vi "UpperMidbrain.vi"(5 "Boat Heading":dbl, 6 "tweak":T2, 7 "WhatAroundMeMap?":cluster{"T":dbl, "Range":dbl, "Bearing":dbl}[](array[cluster]), 8 "SOFT E-STOP":bool, 9 "behavior weights":i8[](array[numeric])=[0, 1, 0], 10 "ir distance":i32, 11 "ForeBrain to Midbrain":T1) -> (3 "string":string)   [LabVIEW 2012]
panel:
  # "under cloud?"
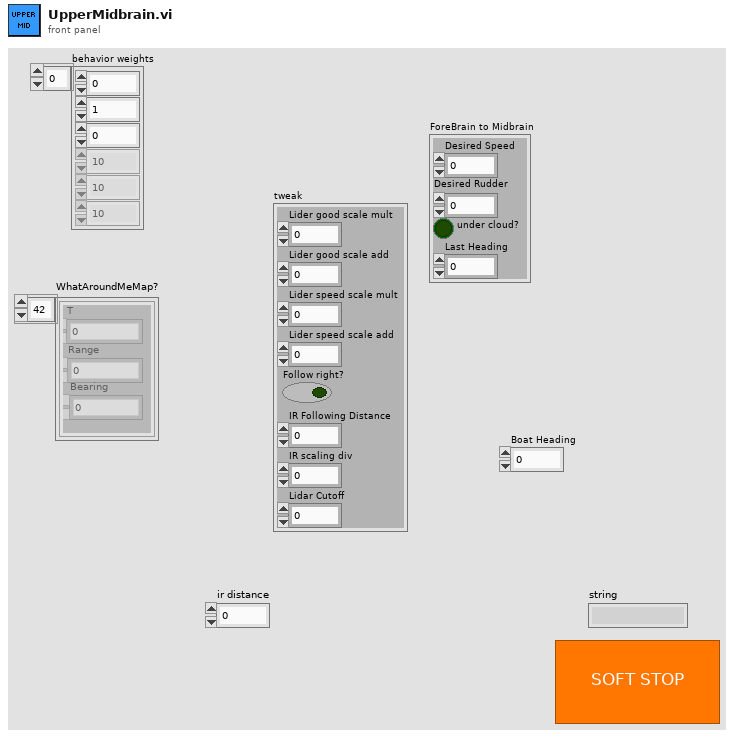
[diagram p1: front panel]
types:
  T1 = cluster{"Desired Speed":i16, "Desired Rudder":i16, bool, "Last Heading":i16}
  T2 = cluster{"Lider good scale mult":dbl, "Lider good scale add":dbl, "Lider speed scale mult":dbl, "Lider speed scale add":dbl, "Follow right?":bool, "IR Following Distance":i32, "IR scaling div":dbl, "Lidar Cutoff":dbl}
  T3 = typedef "behaviorOutput_t.ctl" = cluster{"Goodness":i8[], "Velocity":i8[], "Weight":i8}
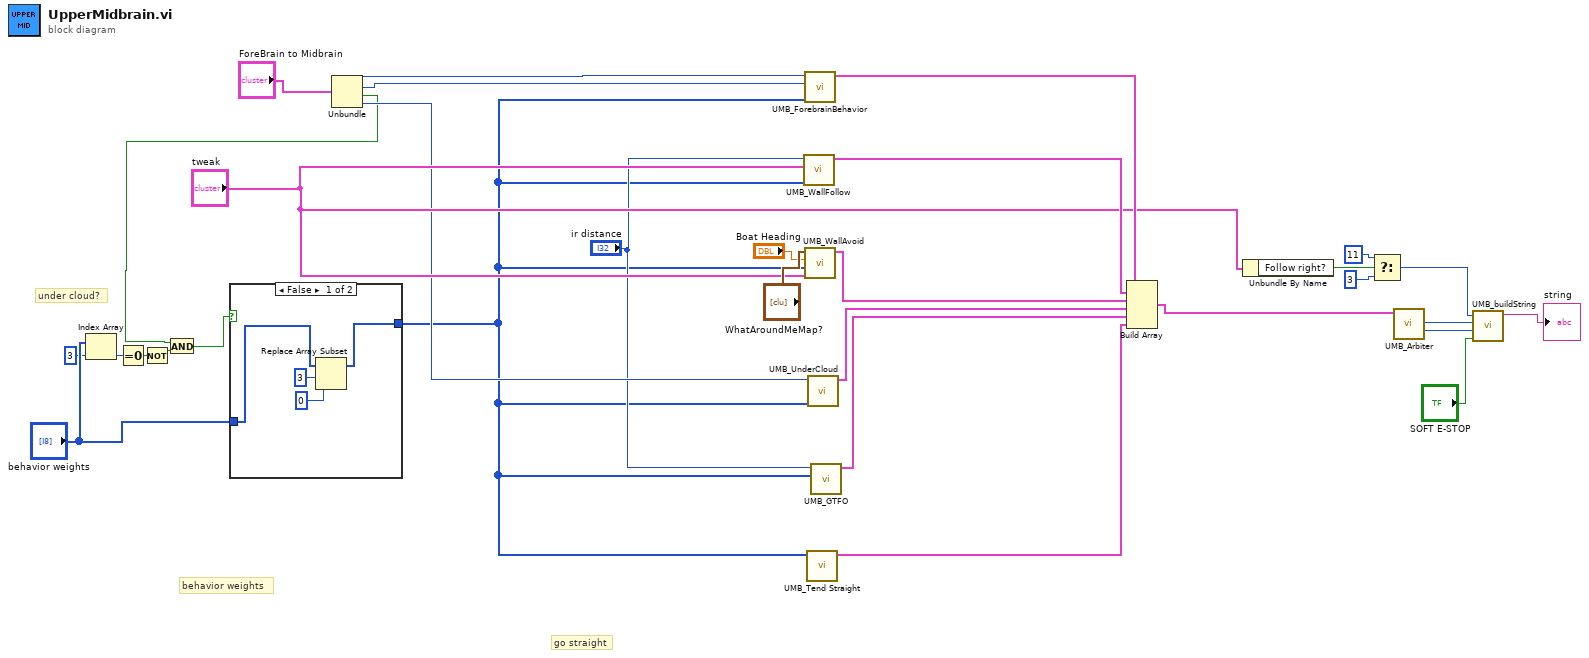
[diagram p0: block diagram]
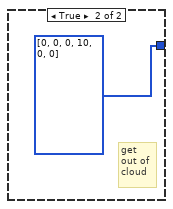
[diagram p2: hidden frame]
diagram:
  # "go straight"
  # "under cloud?"
  # "behavior weights"
  n1 = Index Array(array="behavior weights", index=3) -> (element=w5:i8)
  n2 = Equal To 0?(x=w5) -> (x = 0?=w1:bool)
  n3 = Not(x=w1) -> (.not. x?=w2:bool)
  n4 = Unbundle("ForeBrain to Midbrain") -> ("Desired Speed"=w8:i16, "Desired Rudder"=w16:i16, w4:bool, "Last Heading"=w14:i16)
  n5 = And(x=w4, y=w2) -> (x .and. y?=w3:bool)
  n6 = case shown="False" w3 {
    tunnel: [w33 i8[] [0, 0, 0, 10, 0, 0] ("behavior weights 2")] -> w9
    tunnel: "behavior weights" -> [w34 _]
    frame False {
      n7 = Replace Array Subset(array=w34, new element=i8 0 ("new element/subarray"), index=3) -> (w33:i8[])
    }
    frame True {
      # "get out of cloud"
    }
  }
  n8 = call "UMB_WallFollow.vi"("behavior weights"=w9, "tweak cluster"="tweak", "ir distance"="ir distance") -> ("Behavior Output"=w26:T3)  [unwired: 8 in]
  n9 = call "UMB_ForebrainBehavior.vi"("behavior weights"=w9, "Desired Velocity"=w16, "Desired Heading"=w8) -> ("Behavior Output"=w27:T3)  [unwired: 8 in]
  n10 = call "UMB_WallAvoid.vi"("tweak cluster"="tweak", "behavior weights"=w9, "Boat Heading"="Boat Heading", "WhatAroundMeMap?"="WhatAroundMeMap?") -> ("Behavior Output"=w25:T3)  [unwired: 7 in]
  n11 = call "UMB_Tend Straight.vi"("behavior weights"=w9) -> ("Behavior Output"=w11:T3)  [unwired: 10 in]
  n12 = call "UMB_UnderCloud.vi"("behavior weights"=w9, "Last Heading"=w14) -> ("Behavior Output"=w23:T3)  [unwired: 9 in]
  n13 = call "UMB_GTFO.vi"("behavior weights"=w9, "IR distance"="ir distance") -> ("Behavior Output"=w13:T3)  [unwired: 9 in]
  n14 = Build Array(w27, w26, w25, w23, w13, w11) -> (w28:T3[])
  n15 = Unbundle By Name("tweak") -> ("Follow right?"=w19:bool)
  n16 = Select(t=i8 11, s=w19, f=i8 3) -> (s? t:f=w20:i8)
  n17 = call "UMB_Arbiter.vi"("Behavior Data"=w28) -> ("prop"=w29:i8, "rudder"=w30:i32)  [unwired: 9 in]
  n18 = call "UMB_buildString.vi"("soft e-stop"="SOFT E-STOP", "Prop"=w29, "Rudder"=w30, "IR Servo"=w20) -> ("string"=→"string":string)  [unwired: 7 in]
